vi "Pannello_ElectricalTests.vi"() -> ()   [LabVIEW 2015]
panel:
  in  "New Session":bool
  in  "Stop Button":bool
  in  "Tab Control":T1(tab)
  in  "DONE WITH PCB NAMING?":bool
  in  "DONE WITH BOTH SIDES?":bool
  in  "Punto 1 (MOhm)":string
  in  "Punto 2 (MOhm)":string
  in  "Punto 3 (MOhm)":string
  in  "Punto 4 (MOhm)":string
  in  "Punto 5 (MOhm)":string
  in  "PCB NAME (e.g SE1004)":string
  in  "Punto 1 (MOhm)":string
  in  "Punto 2 (MOhm)":string
  in  "Punto 3 (MOhm)":string
  in  "Punto 4 (MOhm)":string
  in  "Punto 5 (MOhm)":string
  in  "Comment":string
  in  "Punto 9 (MOhm)":string
  in  "Punto 8 (MOhm)":string
  in  "Punto 7 (MOhm)":string
  in  "Punto 6 (MOhm)":string
  in  "Punto 9 (MOhm)":string
  in  "Punto 8 (MOhm)":string
  in  "Punto 7 (MOhm)":string
  in  "Punto 6 (MOhm)":string
  in  "Punto 1 (MOhm)":string
  in  "Punto 2 (MOhm)":string
  in  "Punto 3 (MOhm)":string
  in  "Punto 4 (MOhm)":string
  in  "Punto 5 (MOhm)":string
  in  "Punto 1 (MOhm)":string
  in  "Punto 2 (MOhm)":string
  in  "Punto 3 (MOhm)":string
  in  "Punto 4 (MOhm)":string
  in  "Punto 5 (MOhm)":string
  in  "DONE WITH BOTH SIDES?":bool
  in  "Comment":string
  in  "DX (GOhm)":string
  in  "SX (GOhm)":string
  in  "DONE WITH BOTH SIDES?":bool
  in  "Comment":string
  in  "Meas. 4 (GOhm)":string
  in  "Meas. 3 (GOhm)":string
  in  "DONE WITH BOTH SIDES?":bool
  in  "Meas. 2 (GOhm)":string
  in  "Meas. 1 (GOhm)":string
  in  "Comment":string
  in  "Comment":string
  in  "External (uA)":string
  in  "Internal (uA)":string
  in  "Intermediate (uA)":string
  in  "DONE WITH ALL PCBs?":bool
  # "In this test the resistance of the resistive strips is measured. \nThe measurement is performed between the the resistive strips and the HV.\nThe measurement points are on the borders of the pillar region and the restistive strip contact is achieved through the use of the plexiglass tool probes.\nTools needed: \n- Plexiglass tool with probes\n- Multimeter\n- Two cables with banana plugs\n\nInstructions:\n- Place the electrical tool on one of the PCB sides\n- Connect the first cable on one multimeter pole on one end and on the HV probe on the other\n- Connect the second cable on the other multimeter pole on one end and on one of the 5 resistive strip probes of the other\n- Switch on the multimeter, switch it to the resistance measurement (Ohm) and place it on the table\n- Wait a few seconds until the measurement is stabilized. You should see a value of a few MOhm"
  # "Cu strips"
  # "Silverline"
  # "1"
  # "1"
  # "SX"
  # "SX"
  # "DX"
  # "2"
  # "2"
  # "HV"
  # "HV"
  # "3"
  # "3"
  # "4"
  # "4"
  # "Cu strips"
  # "DX"
  # "5"
  # "5"
  # "In this test the resistance of the resistive strips is measured. \nThe measurement is performed between the resistive strips and the HV.\nThe measurement points are all over the main pillar region and the restistive strip contact is achieved through the use of a single probe (batticarne).\nTools needed: \n- Plexiglass tool with probes\n- Batticarne, plasticized card for the precise positioning of the tool\n- Multimeter\n- Two cables with banana plugs\n\nInstructions:\n- Place the electrical tool on one of the PCB sides\n- Place the plasticized card on the main pillar region in such a way that it is parallel to the PCB sides and close to the plexiglass tool\n- Place the batticarne on point 1 rotated such that the line designed on it and the line of the card hole coincide\n- Connect the first cable on one multimeter pole on one end and on the HV probe on the other\n- Connect the second cable on the other multimeter pole on one end and on the probe of the batticarne\n- Switch on the multimeter, switch it to the resistance measurement (Ohm) and place it on the table\n- Wait a few seconds until the measurement is stabilized. A value of a few MOhm should be obtained."
  # "1"
  # "4"
  # "4"
  # "1"
  # "SX"
  # "DX"
  # "2"
  # "5"
  # "5"
  # "2"
  # "SX"
  # "DX"
  # "3"
  # "6"
  # "6"
  # "3"
  # "In this test the isolation of the silverline due to the coverlay is measured. \nThe measurement is performed between the silverline and the HV.\nThe measurement points are the probe (either of the two) of the silverline and the HV probe.\nThis is a HV measurement so be very careful to NOT touch the board while measuring!\nTools needed: \n- Plexiglass tool with probes\n- Megger\n- Two HV cables with banana plugs\n\nInstructions:\n- Place the electrical tool on one of the PCB sides\n- Open the Megger box and connect the HV cables on the + and - inputs\n- Connect the other end of one of the HV cables on the silverline probe\n- Connect the other end of the second HV on the HV probe\n- MAKE SURE THE HV CABLES ARE CONNECTED TO THE RIGHT PROBES!!! MAKE SURE THERE ARE NO OBJECTS ON THE PCB!\n- Switch on the Megger and set it to 1000V for 2 minutes\n- Move away from the PCB!\n- Start the measurement by keeping pressed the red button until you hear a clicking sound\n- Wait until the measurement ends (Megger light will switch off, and you will hear the clicking sound again)"
  # "Here you should see a value of above 300 GOhm."
  # "In this test the isolation of the Cu strips from the resistive strips due to the kapton layer is measured. \nThe measurement is performed between the HV and Cu strips.\nThe measurement points are the HV probe (or the batticarne probe) and the Cu strip probe.\nThis is a HV measurement so be very careful to NOT touch the board while measuring!\nTools needed: \n- Plexiglass tool with probes\n- Megger\n- Batticarne\n- Two HV cables with banana plugs\n\nInstructions:\nSince the resistive strips are cut in the middle of the PCB (left from right) and the Cu strips are divided into two sides (up and down), there \nare 4 measurements to be performed.\n- Measurement 1: HV probe vs. Cu strips (top right PCB part)\n- Measurement 2: Batticarne probe vs. Cu strips (top left PCB part)\n- Measurement 3: HV probe vs. Cu strips (bottom left PCB part)\n- Measurement 4: Batticarne probe vs. Cu strips (bottom right PCB part)"
  # "Here you should see a value of above 13 GOhm."
  # "SX"
  # "DX"
  # "In this test the current drawn in high electrical potential is measured. For this reason the two mesh tools are placed on the PCBs pillar zone,\nthey are shorted (black cable) and connected to the \"-\" contact of the Megger. The PCB HV lines are also shorted (red cable, red connector) and connected to the \"+\" contact of the Megger.\nThis is a HV measurement so be very careful to NOT touch the board while measuring!\nTools needed: \n- Two mesh tools\n- Black banana cable\n- Red banana HV cable\n- Red HV connector\n- Megger\n\nInstructions:\nHere the current is measurered, so first select the current (I) indication on the right side of the Megger display. Each measurement is performed at 625V for 5'. During the first seocnds of the measurement\na current of the level of a few uA is drawn, which slowly drops to a few hundreds of nA once 5' have elapsed. The measurement points depend on the size of the PCB and are selected in such a way so as to \ncover as much as the active area is possible:\n- PCB 1: One measurement (fill the \"external\" slot only)\n- PCB 2: Two measurements, \"internal\" and \"external\"\n- PCB 3: Two measurements, \"internal\" and \"external\"\n- PCB 4: Three measurements, \"internal\", \"intermediate\" and \"external\"\n- PCB 3: Three measurements, \"internal\", \"intermediate\" and \"external\""
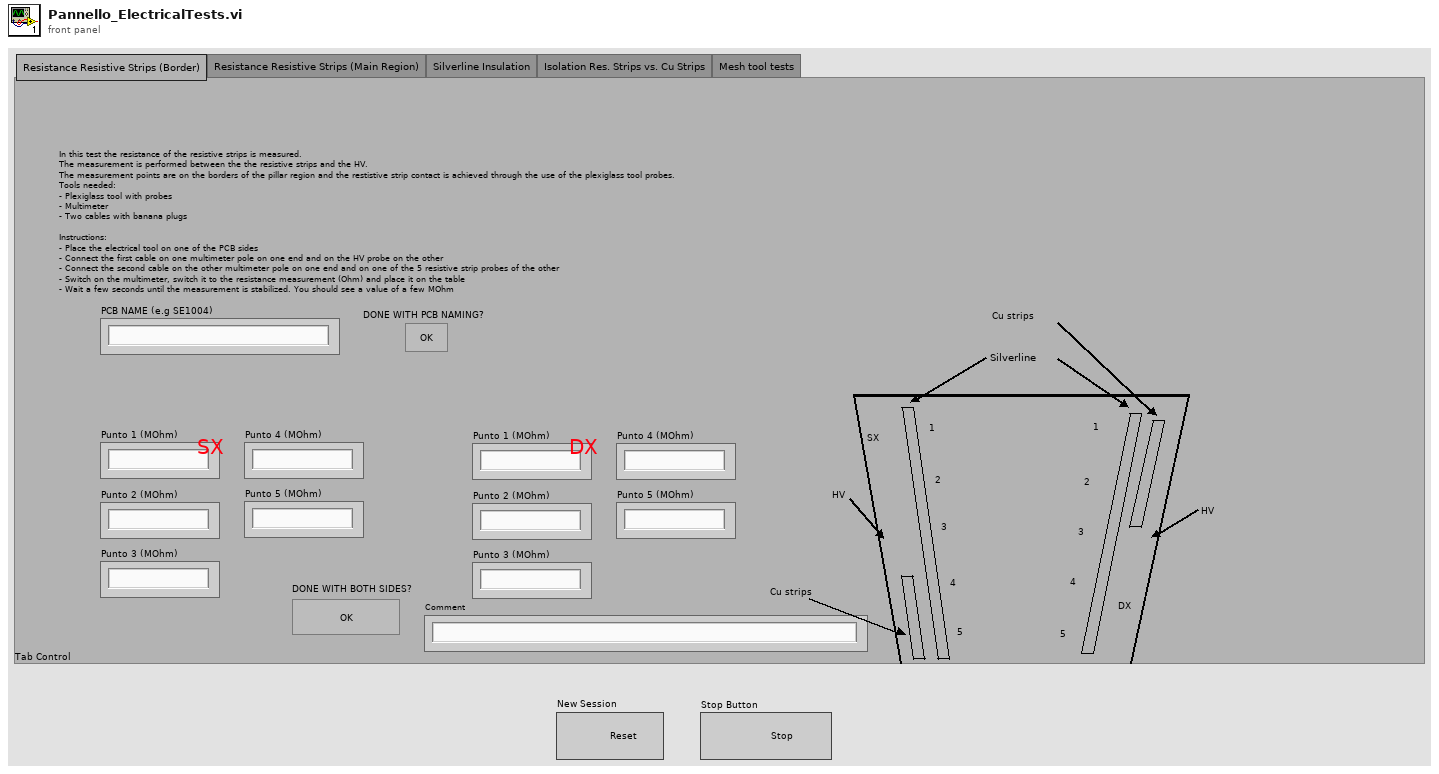
[diagram p1: front panel]
types:
  T1 = enum32{"Resistance Resistive Strips (Border)", "Resistance Resistive Strips (Main Region)", "Silverline Insulation", "Isolation Res. Strips vs. Cu Strips", "Mesh tool tests"}
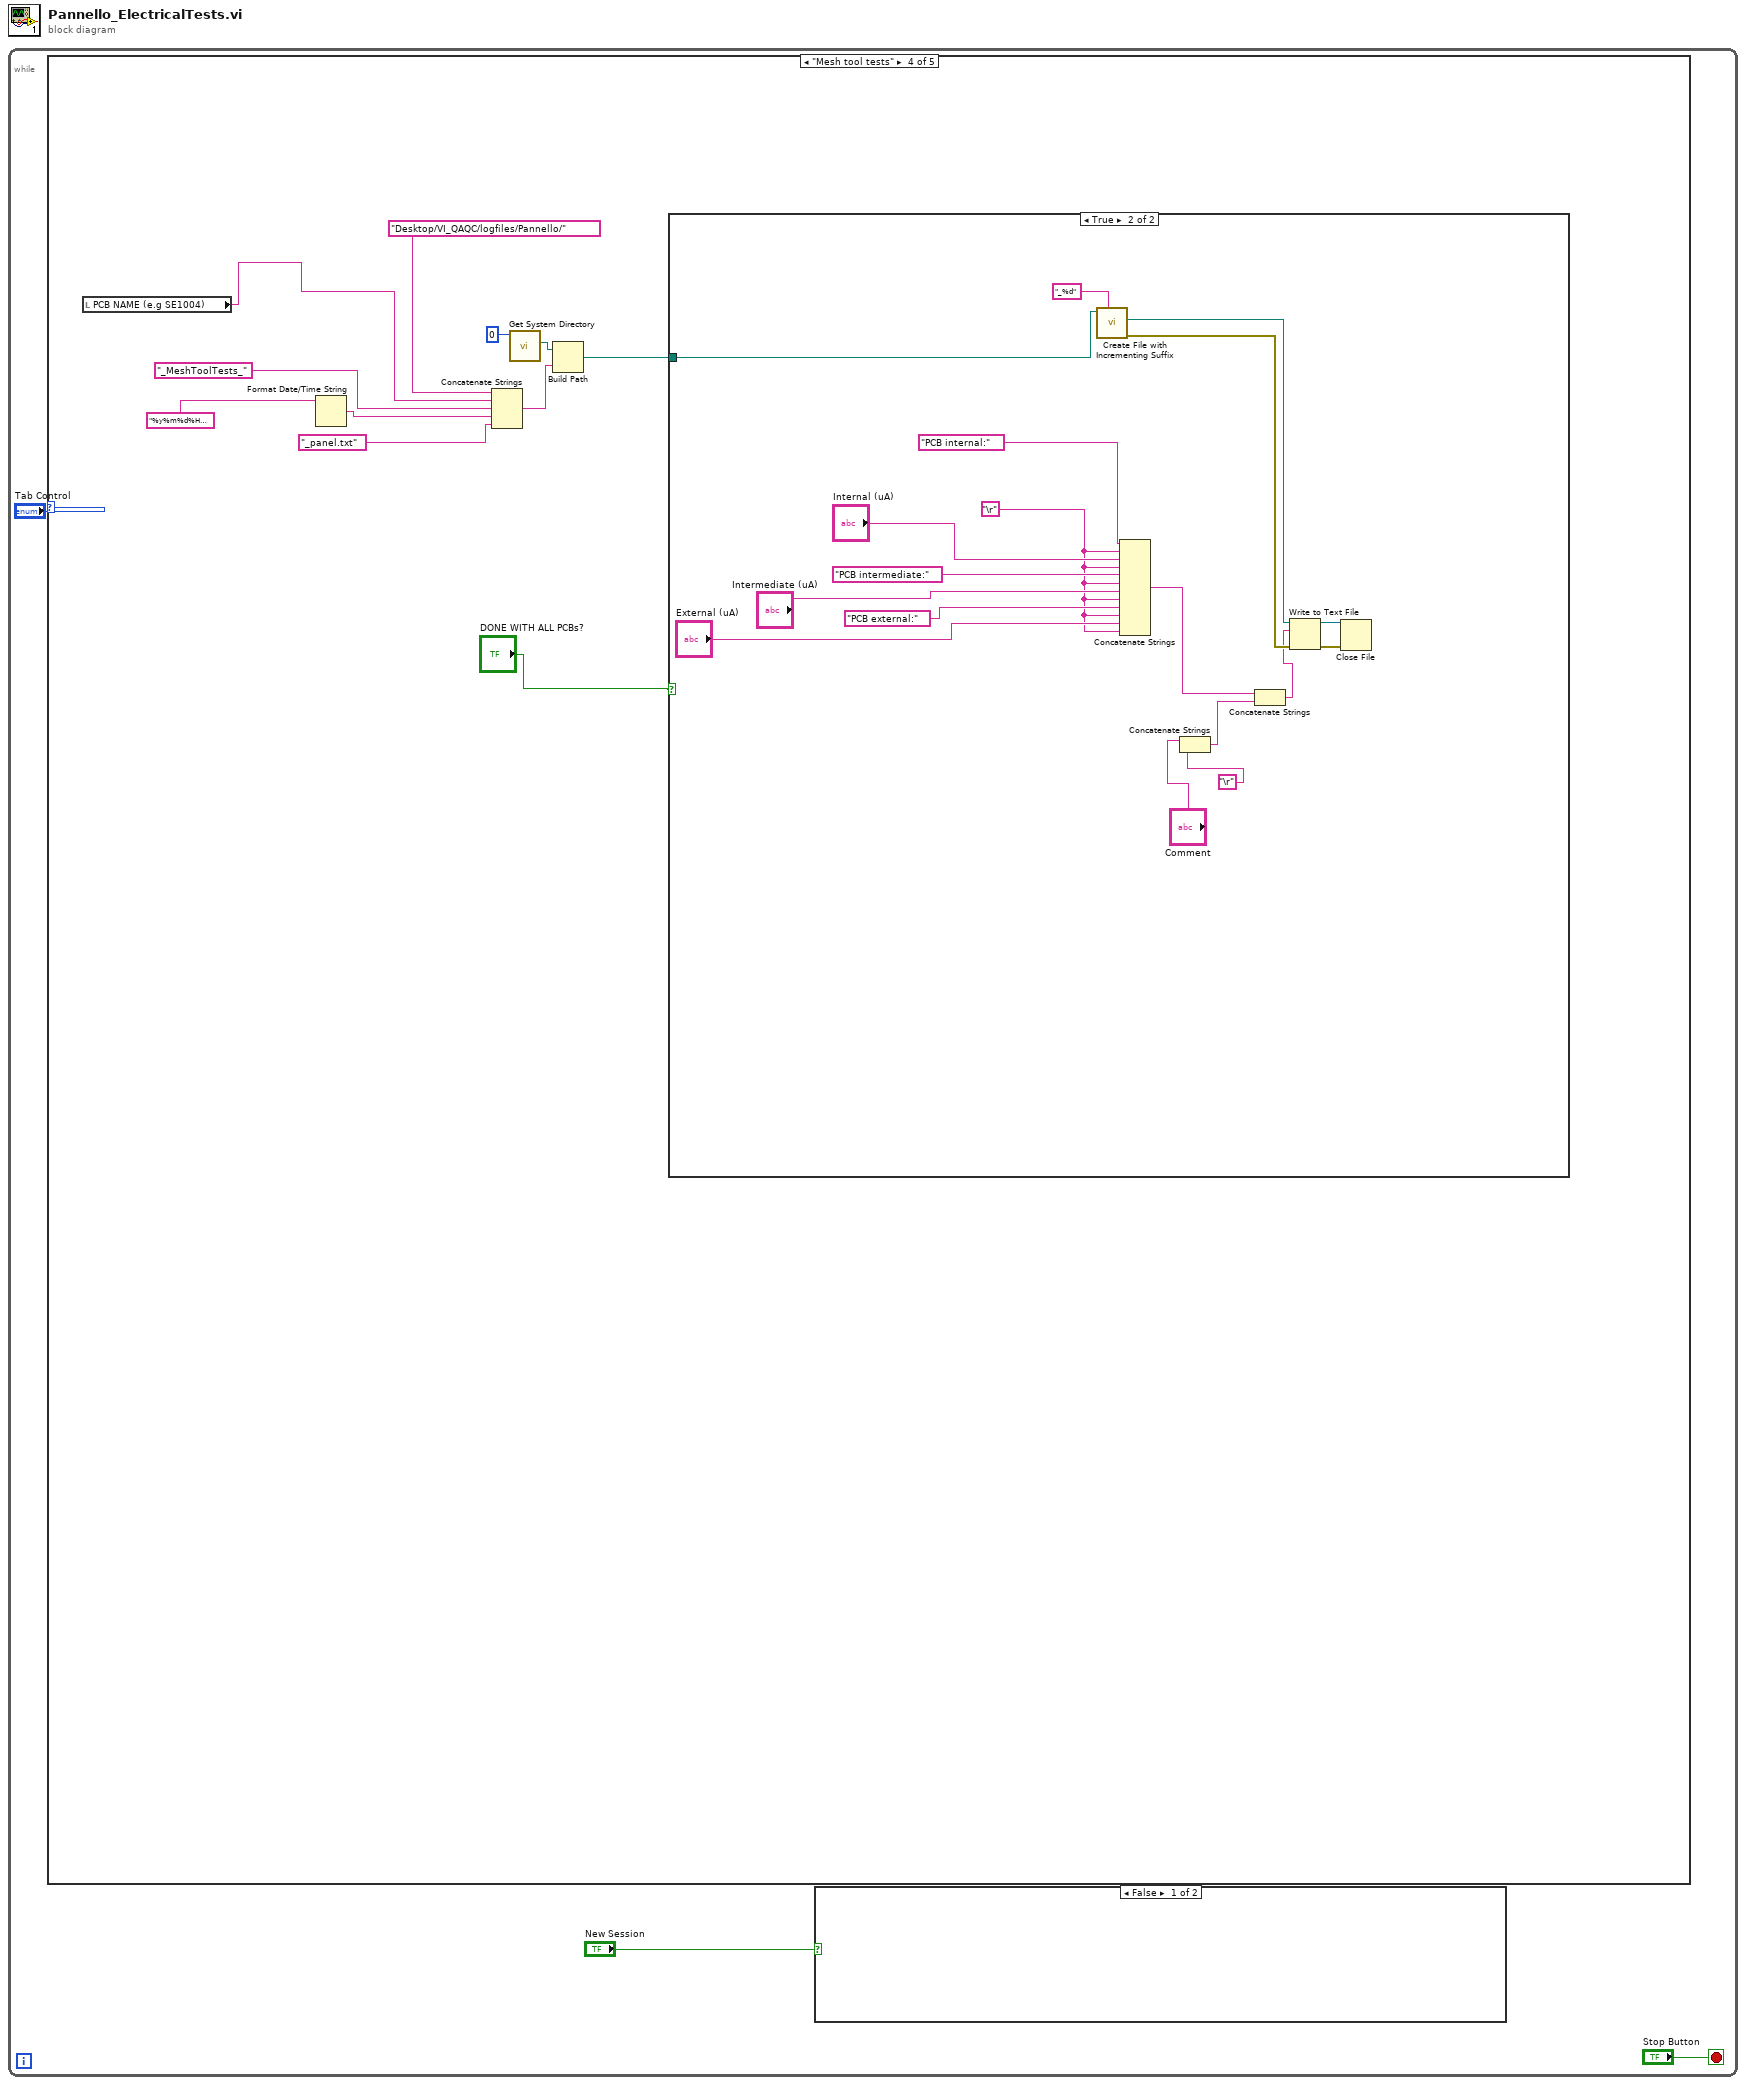
[diagram p0: block diagram]
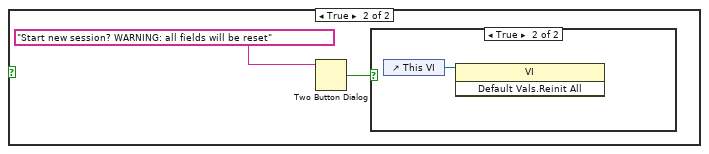
[diagram p2: hidden frame]
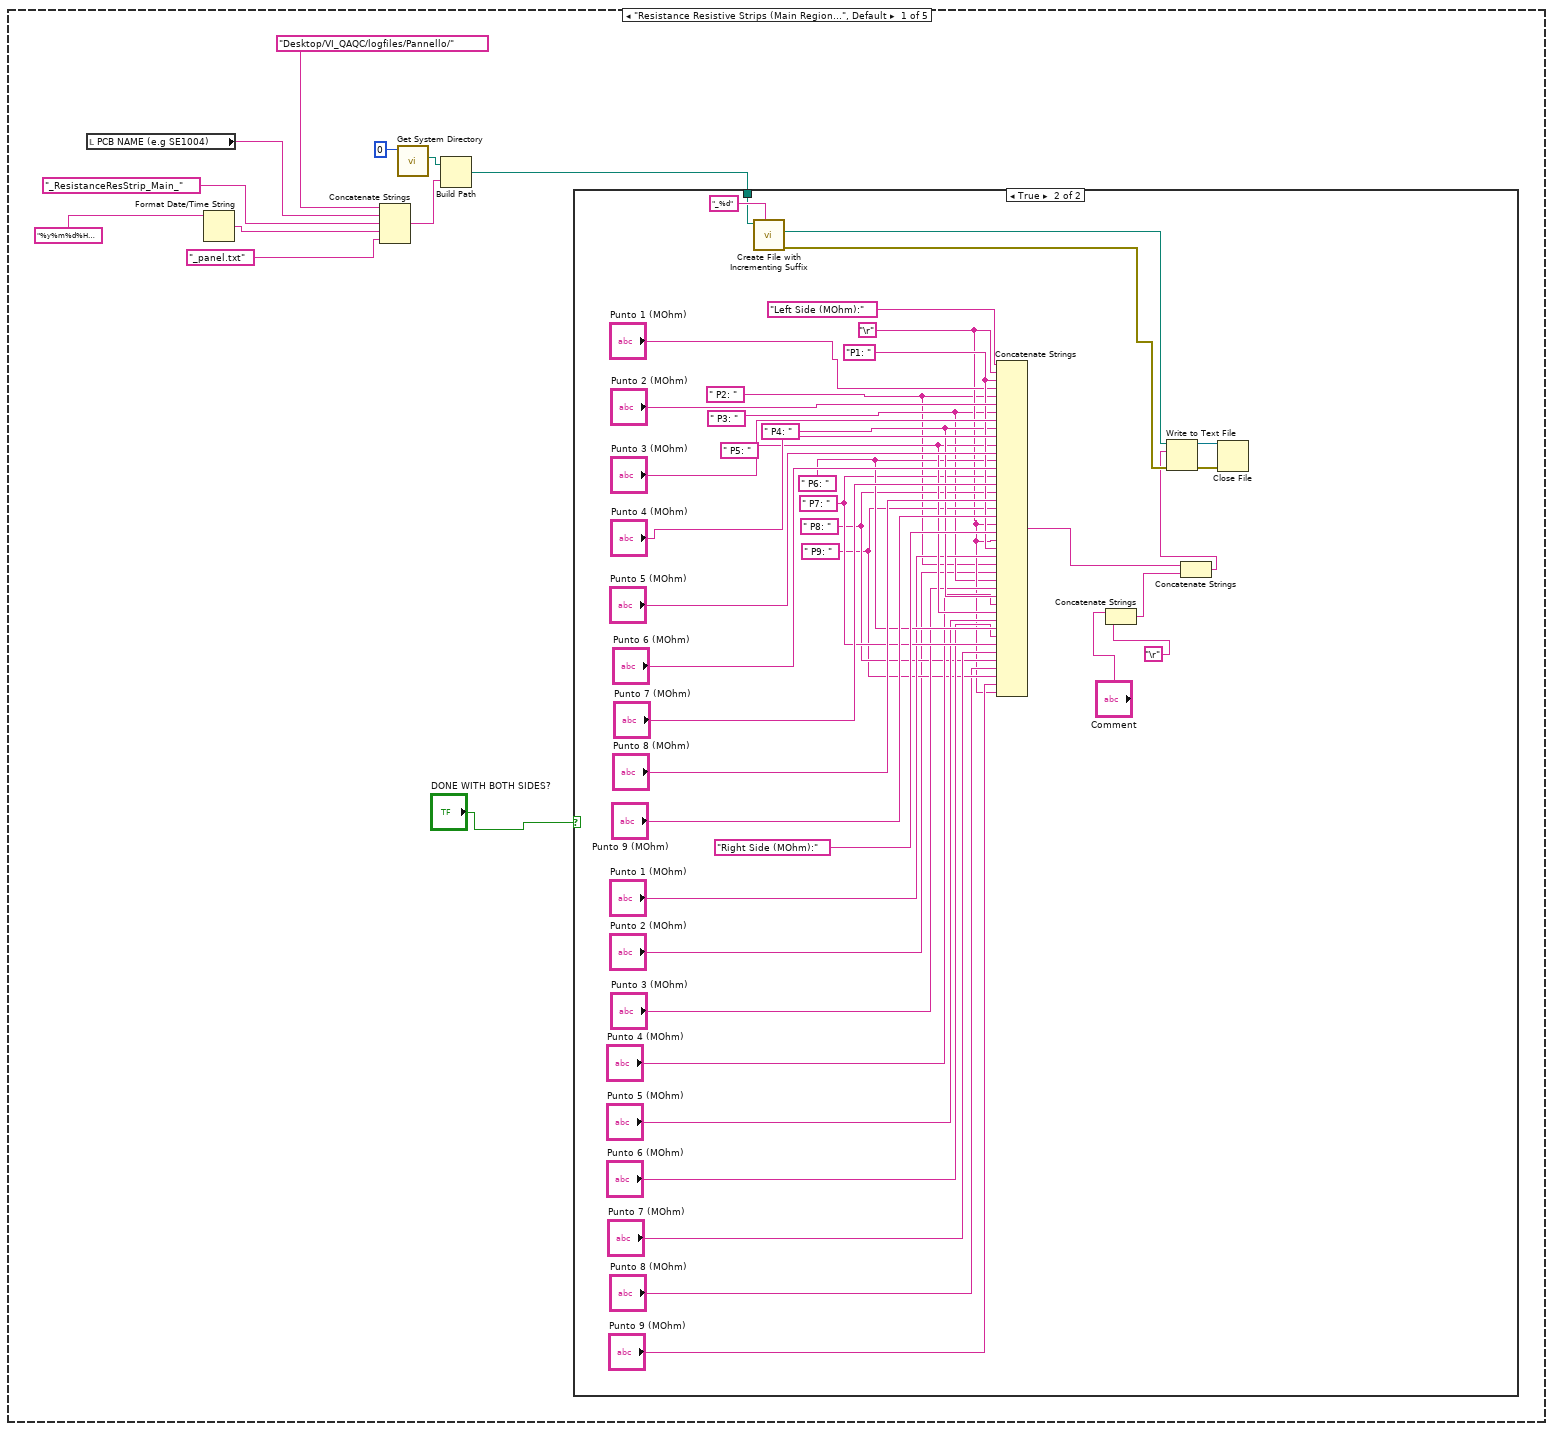
[diagram p4: hidden frame]
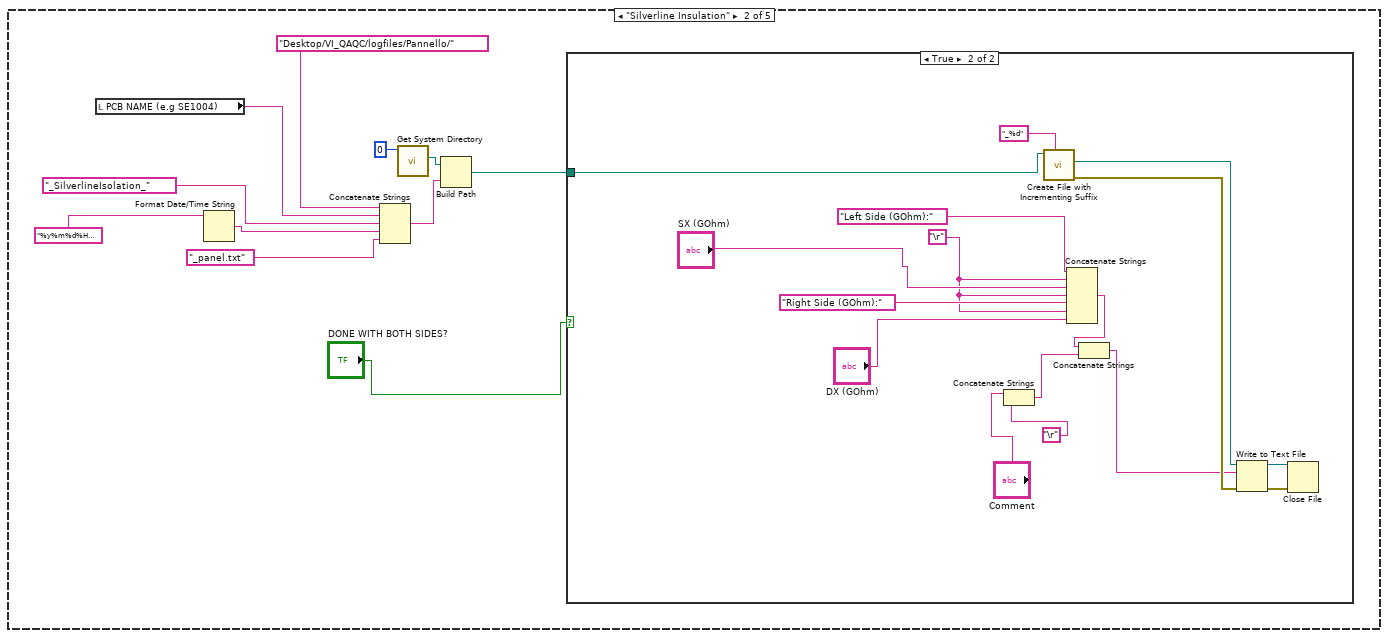
[diagram p6: hidden frame]
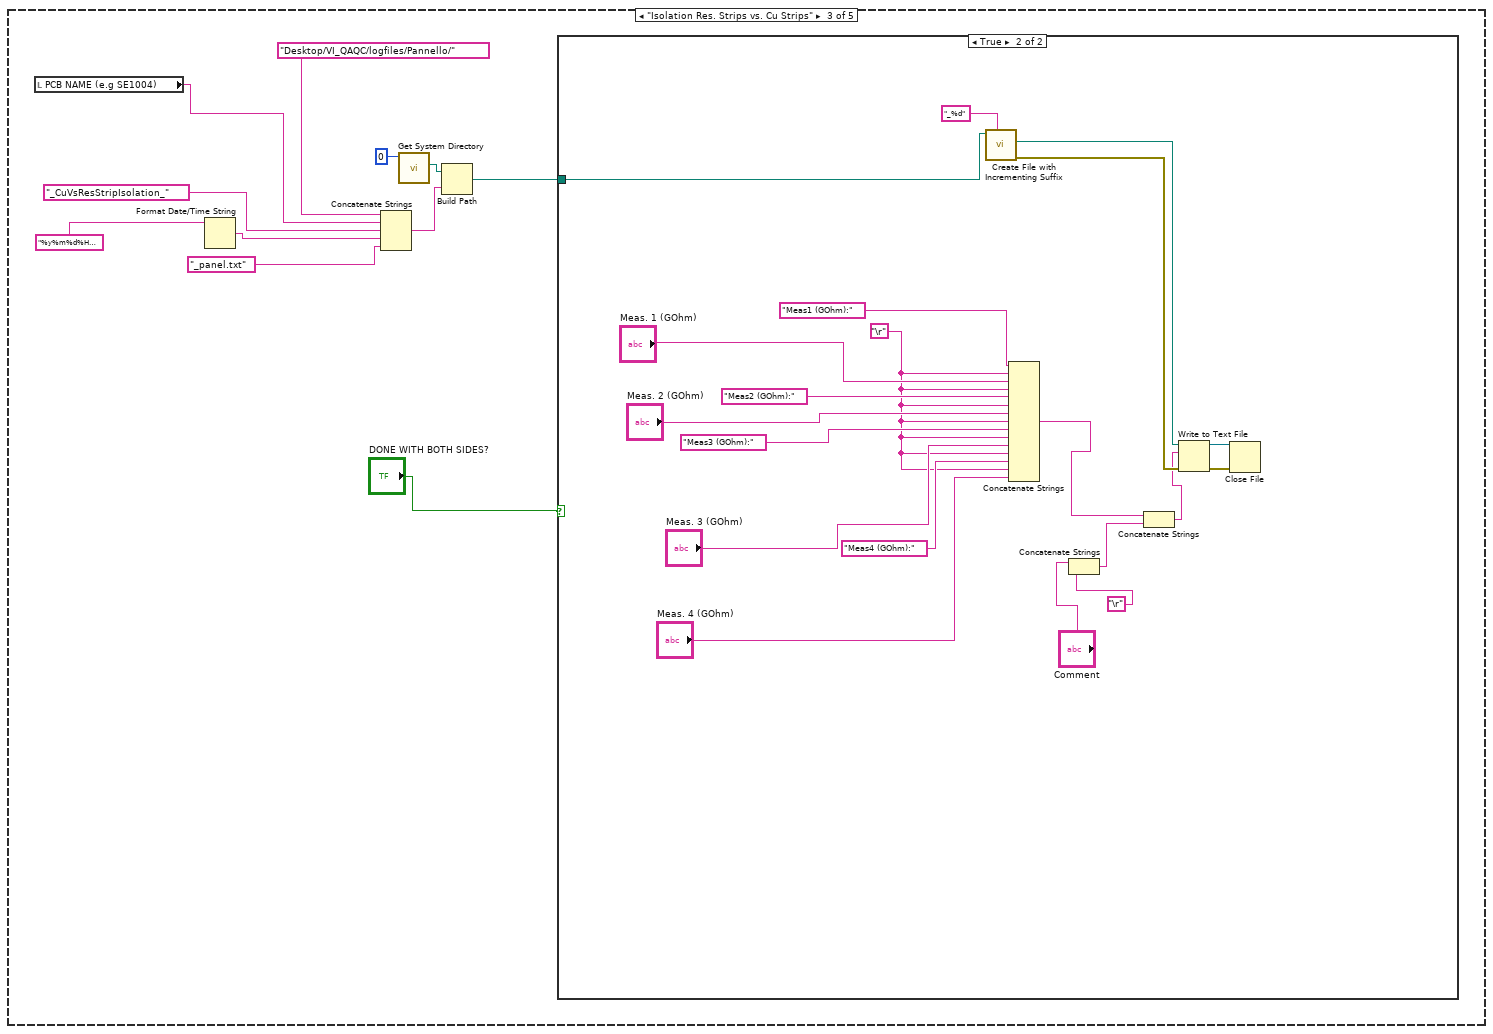
[diagram p8: hidden frame]
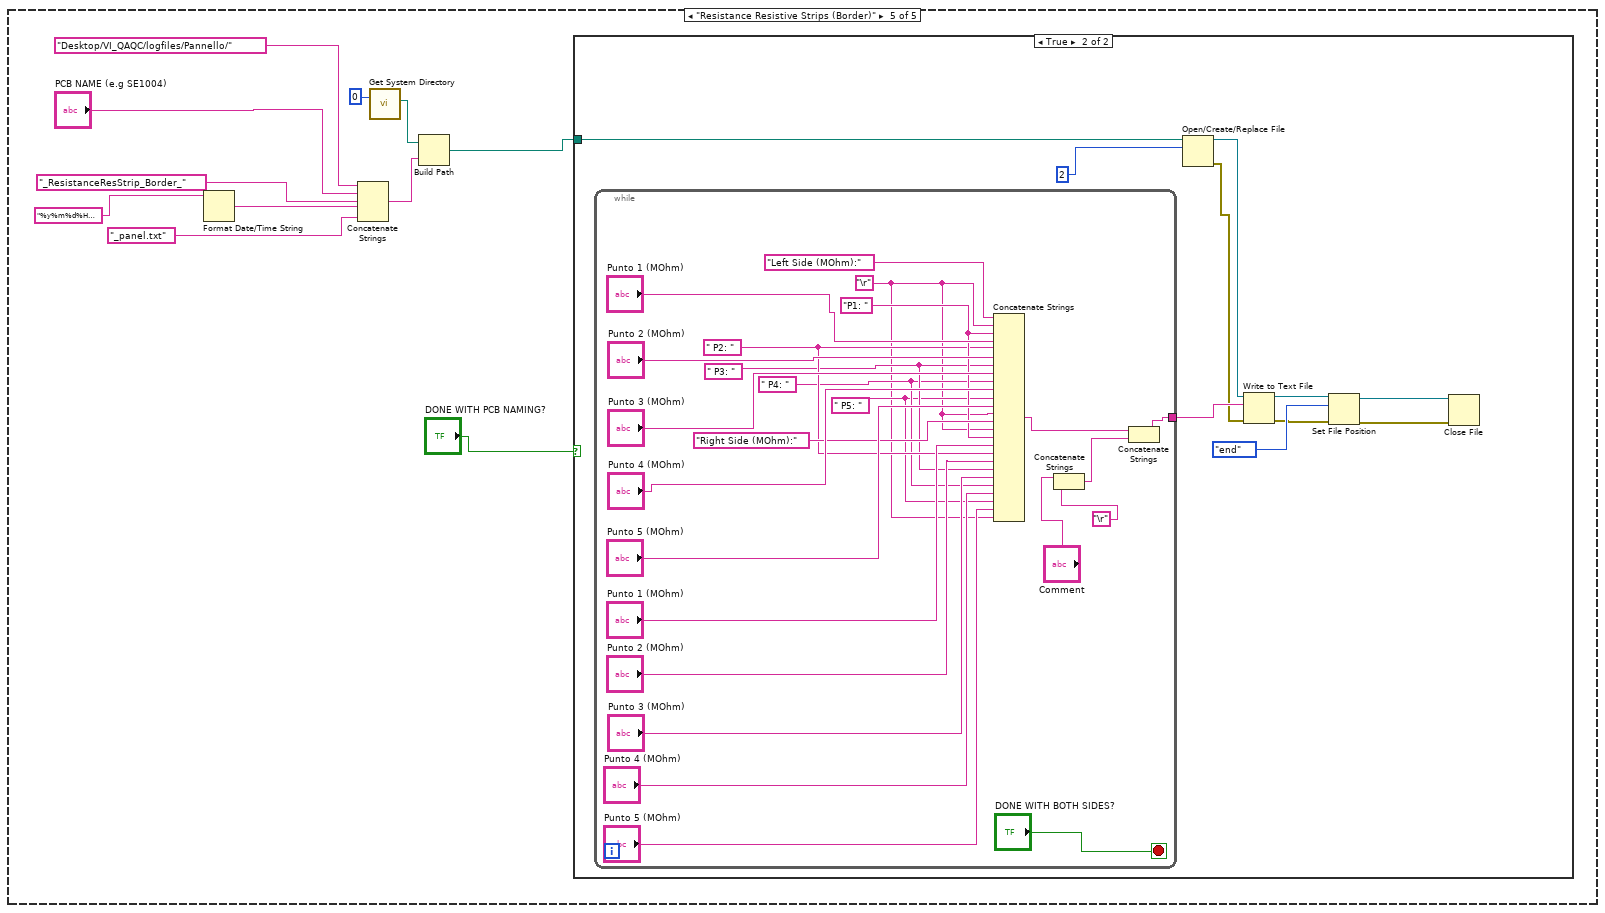
[diagram p11: hidden frame]
diagram:
  n1 = while {
    stop <- "Stop Button" stop-if-true
    n2 = case shown="\"Mesh tool tests\"" "Tab Control" {
      frame "Resistance Resistive Strips (Main Region)", Default {
        n3 = local read "PCB NAME (e.g SE1004)"() -> (w9:string)
        n4 = Format Date/Time String(time format string (%c)="%y%m%d%H%M") -> (date/time string=w10:string)  [unwired: 2 in]
        n5 = Concatenate Strings("Desktop/VI_QAQC/logfiles/Pannello/", w9, "_ResistanceResStrip_Main_", w10, "_panel.txt") -> (w15:string)
        n6 = call <vilib>:"Get System Directory.vi"("system directory type"=0) -> ("system directory"=w16:path)  [unwired: 10 in]
        n7 = Build Path(base path=w16, name or relative path=w15) -> (appended path=w7:path)
        n8 = case shown="True" "DONE WITH BOTH SIDES?" {
          tunnel: w7 -> [_ w28]
          frame False {
          }
          frame True {
            w33 = " P9: "
            w34 = " P8: "
            w41 = " P7: "
            w42 = " P6: "
            w43 = " P5: "
            w44 = " P4: "
            w25 = " P3: "
            w23 = " P2: "
            w46 = "P1: "
            w30 = "\r"
            n9 = call <vilib>:"Create File with Incrementing Suffix.vi"("format string (\" (%d)\")"="_%d" ("format string (\" (%d)\")"), "file path"=w28) -> ("error out"=w27:errorcluster, "actual path"=w26:path)  [unwired: 7 in, 1 out]
            n10 = Concatenate Strings("Left Side (MOhm):", w30, w46, "Punto 1 (MOhm)", w23, "Punto 2 (MOhm)", w25, "Punto 3 (MOhm)", w44, "Punto 4 (MOhm)", w43, "Punto 5 (MOhm)", w42, "Punto 6 (MOhm)", w41, "Punto 7 (MOhm)", w34, "Punto 8 (MOhm)", w33, "Punto 9 (MOhm)", w30, "Right Side (MOhm):", w30, w46, "Punto 1 (MOhm)", w23, "Punto 2 (MOhm)", w25, "Punto 3 (MOhm)", w44, "Punto 4 (MOhm)", w43, "Punto 5 (MOhm)", w42, "Punto 6 (MOhm)", w41, "Punto 7 (MOhm)", w34, "Punto 8 (MOhm)", w33, "Punto 9 (MOhm)", w30) -> (w19:string)
            n11 = Concatenate Strings("Comment", "\r") -> (w20:string)
            n12 = Concatenate Strings(w19, w20) -> (w18:string)
            n13 = Write to Text File(file (use dialog)=w26, text=w18, error in=w27) -> (refnum out=w57:refnum<file>, error out=w58:errorcluster)  [unwired: 1 in, 1 out]
            n14 = Close File(refnum=w57, error in=w58) -> ()  [unwired: 2 out]
          }
        }
      }
      frame "Silverline Insulation" {
        n15 = local read "PCB NAME (e.g SE1004)"() -> (w60:string)
        n16 = Format Date/Time String(time format string (%c)="%y%m%d%H%M") -> (date/time string=w61:string)  [unwired: 2 in]
        n17 = Concatenate Strings("Desktop/VI_QAQC/logfiles/Pannello/", w60, "_SilverlineIsolation_", w61, "_panel.txt") -> (w67:string)
        n18 = call <vilib>:"Get System Directory.vi"("system directory type"=0) -> ("system directory"=w68:path)  [unwired: 10 in]
        n19 = Build Path(base path=w68, name or relative path=w67) -> (appended path=w66:path)
        n20 = case shown="True" "DONE WITH BOTH SIDES?" {
          tunnel: w66 -> [_ w82]
          frame False {
          }
          frame True {
            w76 = "\r"
            n21 = Concatenate Strings("Comment", "\r") -> (w72:string)
            n22 = call <vilib>:"Create File with Incrementing Suffix.vi"("format string (\" (%d)\")"="_%d" ("format string (\" (%d)\")"), "file path"=w82) -> ("error out"=w80:errorcluster, "actual path"=w81:path)  [unwired: 7 in, 1 out]
            n23 = Concatenate Strings("Left Side (GOhm):", w76, "SX (GOhm)", w76, "Right Side (GOhm):", w76, "DX (GOhm)") -> (w71:string)
            n24 = Concatenate Strings(w71, w72) -> (w70:string)
            n25 = Write to Text File(file (use dialog)=w81, text=w70, error in=w80) -> (refnum out=w84:refnum<file>, error out=w85:errorcluster)  [unwired: 1 in, 1 out]
            n26 = Close File(refnum=w84, error in=w85) -> ()  [unwired: 2 out]
          }
        }
      }
      frame "Isolation Res. Strips vs. Cu Strips" {
        n27 = local read "PCB NAME (e.g SE1004)"() -> (w87:string)
        n28 = Format Date/Time String(time format string (%c)="%y%m%d%H%M") -> (date/time string=w88:string)  [unwired: 2 in]
        n29 = Concatenate Strings("Desktop/VI_QAQC/logfiles/Pannello/", w87, "_CuVsResStripIsolation_", w88, "_panel.txt") -> (w94:string)
        n30 = call <vilib>:"Get System Directory.vi"("system directory type"=0) -> ("system directory"=w95:path)  [unwired: 10 in]
        n31 = Build Path(base path=w95, name or relative path=w94) -> (appended path=w93:path)
        n32 = case shown="True" "DONE WITH BOTH SIDES?" {
          tunnel: w93 -> [_ w113]
          frame False {
          }
          frame True {
            w103 = "\r"
            n33 = call <vilib>:"Create File with Incrementing Suffix.vi"("format string (\" (%d)\")"="_%d" ("format string (\" (%d)\")"), "file path"=w113) -> ("error out"=w111:errorcluster, "actual path"=w112:path)  [unwired: 7 in, 1 out]
            n34 = Concatenate Strings("Meas1 (GOhm):", w103, "Meas. 1 (GOhm)", w103, "Meas2 (GOhm):", w103, "Meas. 2 (GOhm)", w103, "Meas3 (GOhm):", w103, "Meas. 3 (GOhm)", w103, "Meas4 (GOhm):", w103, "Meas. 4 (GOhm)") -> (w98:string)
            n35 = Concatenate Strings("Comment", "\r") -> (w99:string)
            n36 = Concatenate Strings(w98, w99) -> (w97:string)
            n37 = Write to Text File(file (use dialog)=w112, text=w97, error in=w111) -> (refnum out=w115:refnum<file>, error out=w116:errorcluster)  [unwired: 1 in, 1 out]
            n38 = Close File(refnum=w115, error in=w116) -> ()  [unwired: 2 out]
          }
        }
      }
      frame "Mesh tool tests" {
        n39 = local read "PCB NAME (e.g SE1004)"() -> (w117:string)
        n40 = Format Date/Time String(time format string (%c)="%y%m%d%H%M") -> (date/time string=w119:string)  [unwired: 2 in]
        n41 = Concatenate Strings("Desktop/VI_QAQC/logfiles/Pannello/", w117, "_MeshToolTests_", w119, "_panel.txt") -> (w125:string)
        n42 = call <vilib>:"Get System Directory.vi"("system directory type"=0) -> ("system directory"=w126:path)  [unwired: 10 in]
        n43 = Build Path(base path=w126, name or relative path=w125) -> (appended path=w124:path)
        n44 = case shown="True" "DONE WITH ALL PCBs?" {
          tunnel: w124 -> [_ w142]
          frame False {
          }
          frame True {
            w128 = "\r"
            n45 = call <vilib>:"Create File with Incrementing Suffix.vi"("format string (\" (%d)\")"="_%d" ("format string (\" (%d)\")"), "file path"=w142) -> ("error out"=w140:errorcluster, "actual path"=w141:path)  [unwired: 7 in, 1 out]
            n46 = Concatenate Strings("PCB internal:", w128, "Internal (uA)", w128, "PCB intermediate:", w128, "Intermediate (uA)", w128, "PCB external:", w128, "External (uA)", w128) -> (w133:string)
            n47 = Concatenate Strings("Comment", "\r") -> (w134:string)
            n48 = Concatenate Strings(w133, w134) -> (w132:string)
            n49 = Write to Text File(file (use dialog)=w141, text=w132, error in=w140) -> (refnum out=w144:refnum<file>, error out=w145:errorcluster)  [unwired: 1 in, 1 out]
            n50 = Close File(refnum=w144, error in=w145) -> ()  [unwired: 2 out]
          }
        }
      }
      frame "Resistance Resistive Strips (Border)" {
        n51 = Format Date/Time String(time format string (%c)="%y%m%d%H%M") -> (date/time string=w149:string)  [unwired: 2 in]
        n52 = Concatenate Strings("Desktop/VI_QAQC/logfiles/Pannello/", "PCB NAME (e.g SE1004)", "_ResistanceResStrip_Border_", w149, "_panel.txt") -> (w154:string)
        n53 = call <vilib>:"Get System Directory.vi"("system directory type"=0) -> ("system directory"=w155:path)  [unwired: 10 in]
        n54 = Build Path(base path=w155, name or relative path=w154) -> (appended path=w148:path)
        n55 = case shown="True" "DONE WITH PCB NAMING?" {
          tunnel: w148 -> [_ w165]
          frame False {
          }
          frame True {
            n56 = while {
              tunnel: [w169] -> w166
              stop <- "DONE WITH BOTH SIDES?" stop-if-true
              w175 = " P5: "
              w177 = " P4: "
              w179 = " P3: "
              w181 = " P2: "
              w183 = "P1: "
              w173 = "\r"
              n57 = Concatenate Strings("Left Side (MOhm):", w173, w183, "Punto 1 (MOhm)", w181, "Punto 2 (MOhm)", w179, "Punto 3 (MOhm)", w177, "Punto 4 (MOhm)", w175, "Punto 5 (MOhm)", w173, "Right Side (MOhm):", w173, w183, "Punto 1 (MOhm)", w181, "Punto 2 (MOhm)", w179, "Punto 3 (MOhm)", w177, "Punto 4 (MOhm)", w175, "Punto 5 (MOhm)", w173) -> (w168:string)
              n58 = Concatenate Strings("Comment", "\r") -> (w167:string)
              n59 = Concatenate Strings(w168, w167) -> (w169:string)
            }
            n60 = Open/Create/Replace File(file path (use dialog)=w165, operation (0:open)=2) -> (refnum out=w163:refnum<file>, error out=w164:errorcluster)  [unwired: 4 in, 1 out]
            n61 = Write to Text File(file (use dialog)=w163, text=w166, error in=w164) -> (refnum out=w160:refnum<file>, error out=w158:errorcluster)  [unwired: 1 in, 1 out]
            n62 = Set File Position(offset (in bytes) (0)=enum16{"end"}."end", refnum=w160, error in=w158) -> (refnum out=w159:refnum<file>, error out=w157:errorcluster)  [unwired: 1 in]
            n63 = Close File(refnum=w159, error in=w157) -> ()  [unwired: 2 out]
          }
        }
      }
    }
    n64 = case shown="False" "New Session" {
      frame False {
      }
      frame True {
        n65 = Two Button Dialog(message="Start new session? WARNING: all fields will be reset") -> (T button?=w4:bool)  [unwired: 2 in]
        n66 = case shown="True" w4 {
          frame False {
          }
          frame True {
            n67 = control-ref of="This VI"() -> (w6:refnum<vi>)
            n68 = invoke class="VI" method="Default Vals.Reinit All"(reference=w6) -> ()  [unwired: 2 in, 3 out]
          }
        }
      }
    }
  }
